vi "Configure Digital Outputs.vi"(0 "VISA resource name":refnum<visa-resource-name>, 1 "Output Dual Connector (T: Enable)":bool=TRUE, 2 "Output Source (0: dosXLR)":i32(ring) items=["dosXLR", "dosBNC"], 3 "Frame Sync Out Invert (T: Enable)":bool=TRUE, 5 "Output Sampling Rate (0)":i32, 7 "Output Carrier Amp Balance (0)":dbl, 9 "Output Carrier Amp Unbalanced (0)":dbl, 11 "error in (no error)":errorcluster, 12 "Output Num Bits (0)":i32, 13 "Digital Preemphasis (0: dioNoDeem)":i32(ring) items=["dioNoDeem", "dioCD501dB0", "dioCD501dB10", "dioJ17dB0", "dioJ17dB20"]) -> (4 "VISA resource name out":refnum<visa-resource-name>, 15 "error out":errorcluster)   [LabVIEW 2014, in "Stanford Research SR1.lvlib"]
doc: "Configures the basic attributes for the Digital outputs."
uses:
  Stanford Research SR1.lvlib
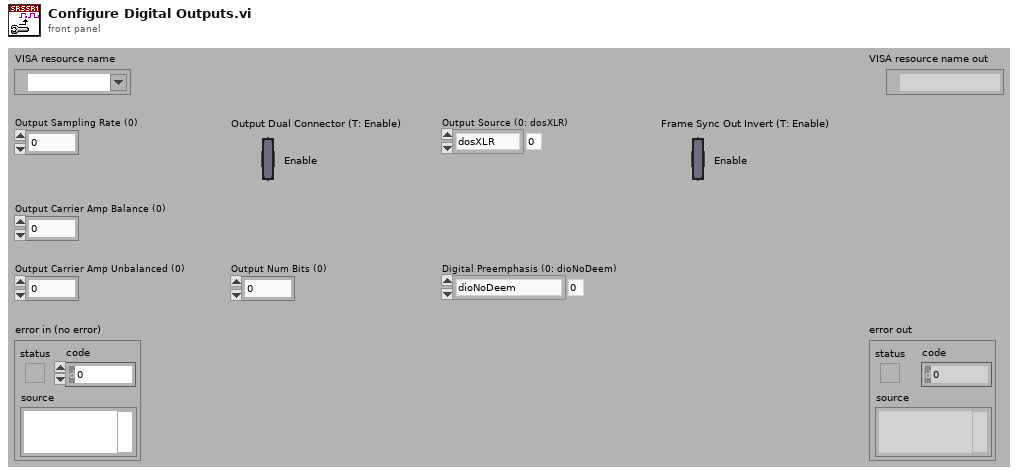
[diagram p1: front panel]
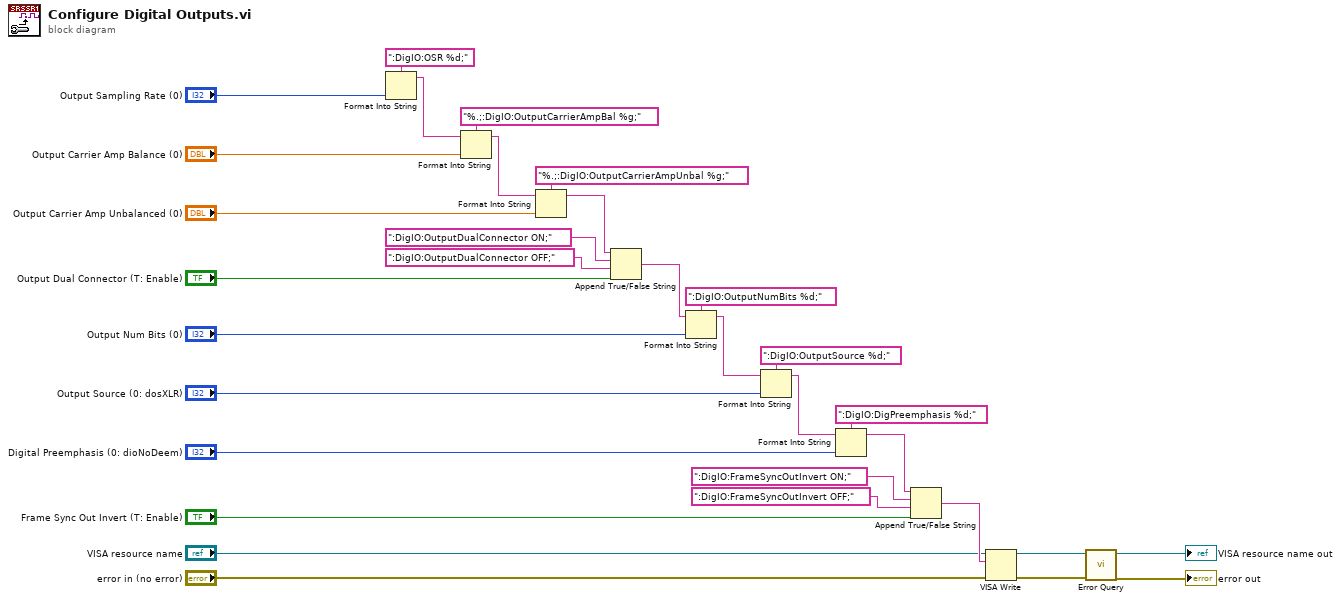
[diagram p0: block diagram]
diagram:
  n1 = Format Into String(format string=":DigIO:OSR %d;", "Output Sampling Rate (0)") -> (resulting string=w30:string)  [unwired: 2 in, 1 out]
  n2 = Format Into String(format string="%.;:DigIO:OutputCarrierAmpBal %g;", initial string=w30, "Output Carrier Amp Balance (0)") -> (resulting string=w27:string)  [unwired: 1 in, 1 out]
  n3 = Format Into String(format string="%.;:DigIO:OutputCarrierAmpUnbal %g;", initial string=w27, "Output Carrier Amp Unbalanced (0)") -> (resulting string=w24:string)  [unwired: 1 in, 1 out]
  n4 = Append True/False String(1:"Output Dual Connector (T: Enable)", 2:":DigIO:OutputDualConnector OFF;", 3:":DigIO:OutputDualConnector ON;", 4:w24) -> (0:w20:string)
  n5 = Format Into String(format string=":DigIO:OutputNumBits %d;", initial string=w20, "Output Num Bits (0)") -> (resulting string=w17:string)  [unwired: 1 in, 1 out]
  n6 = Format Into String(format string=":DigIO:OutputSource %d;", initial string=w17, "Output Source (0: dosXLR)") -> (resulting string=w14:string)  [unwired: 1 in, 1 out]
  n7 = Format Into String(format string=":DigIO:DigPreemphasis %d;", initial string=w14, "Digital Preemphasis (0: dioNoDeem)") -> (resulting string=w11:string)  [unwired: 1 in, 1 out]
  n8 = Append True/False String(1:"Frame Sync Out Invert (T: Enable)", 2:":DigIO:FrameSyncOutInvert OFF;", 3:":DigIO:FrameSyncOutInvert ON;", 4:w11) -> (0:w7:string)
  n9 = VISA Write(VISA resource name="VISA resource name", write buffer=w7, error in (no error)="error in (no error)") -> (VISA resource name out=w4:refnum<visa-resource-name>, error out=w3:errorcluster)  [unwired: 1 out]
  n10 = call "Error Query.vi"("error in (no error)"=w3, "VISA resource name"=w4) -> ("error out"=→"error out":errorcluster, "VISA resource name out"=→"VISA resource name out":refnum<visa-resource-name>)  [unwired: 6 in, 2 out]
